vi "control_PID.vi"() -> ()   [LabVIEW 2022 SP3]
uses:
  <vilib>/Utility/NIReport.llb/Report Type.ctl
  <vilib>/imath/engines/lvmath2/RunTimeEngine/Managers/WorkSpace/UID Generator.vi
  <vilib>/imath/engines/lvmath2/RunTimeEngine/BuiltInFunctions/sin/NIMS_sin(C).vi
  <instcachedir>/0/NIMS_sin(C)_E954A9BB68A349B3841053E554BADAA4.lvgen/NIMS_sin(C)_E954A9BB68A349B3841053E554BADAA4_001.vi
  <vilib>/imath/engines/lvmath2/RunTimeEngine/BuiltInFunctions/cos/NIMS_cos(C).vi
  <instcachedir>/0/NIMS_cos(C)_24E28D29219C4DC6ABC084DC6A0254BF.lvgen/NIMS_cos(C)_24E28D29219C4DC6ABC084DC6A0254BF_001.vi
  <vilib>/imath/engines/lvmath2/RunTimeEngine/BuiltInFunctions/conv/NIMS_conv(V,V).vi
  <instcachedir>/0/NIMS_conv(V,V)_D3E194F2B5174935BB2368CEB7AAC5A9.lvgen/NIMS_conv(V,V)_D3E194F2B5174935BB2368CEB7AAC5A9_000.vi
  <vilib>/imath/engines/lvmath2/RunTimeEngine/ErrorHandling/NIMS_Error From Error Code.vi
  <vilib>/imath/engines/lvmath2/RunTimeEngine/RunTimeType/NIMS_RunTimeType_From StrictType (excl LVString).vi
  <instcachedir>/0/NIMS_RunTimeType_From StrictType (excl LVString)_70DEE8F51B6B495C85F505DE4E7061F1.lvgen/NIMS_RunTimeType_From StrictType (excl LVString)_70DEE8F51B6B495C85F505DE4E7061F1_000.vi
  <vilib>/imath/engines/lvmath2/RunTimeEngine/LocalVariableDefStatement/MC_LocalVariableDefStatement_Display.vi
  <vilib>/imath/engines/lvmath2/RunTimeEngine/IndexRead/NIMS V(S).vi
  <instcachedir>/0/NIMS V(S)_0488751826AF41519A22953C041130DC.lvgen/NIMS V(S)_0488751826AF41519A22953C041130DC_003.vi
  <vilib>/imath/engines/lvmath2/RunTimeEngine/ErrorHandling/NIMS_Create Error From Enums.vi
  <vilib>/imath/engines/lvmath2/RunTimeEngine/BuiltInFunctions/inv/NIMS_inv(GM).vi
  <instcachedir>/0/NIMS_inv(GM)_A6DF8FE880224208AACFE4CF9F659502.lvgen/NIMS_inv(GM)_A6DF8FE880224208AACFE4CF9F659502_001.vi
  <vilib>/imath/engines/lvmath2/RunTimeEngine/ArithmeticOperatorToken/NIMS_ArithmeticOperator_multmx(M,CV).vi
  <instcachedir>/0/NIMS_ArithmeticOperator_multmx(M,CV)_F5DBFFF0126A4383B39F7B34D5ABA6C8.lvgen/NIMS_ArithmeticOperator_multmx(M,CV)_F5DBFFF0126A4383B39F7B34D5ABA6C8_002.vi
  <vilib>/imath/engines/lvmath2/RunTimeEngine/IndexRead/NIMS M(S).vi
  <instcachedir>/0/NIMS M(S)_B826C018497E4940AE96BD27B540B6FB.lvgen/NIMS M(S)_B826C018497E4940AE96BD27B540B6FB_004.vi
  <vilib>/imathl/engines/lvmath/Functions/Error Handling/Create Error.vi
  <vilib>/imath/engines/lvmath2/RunTimeEngine/Managers/SymbolTable/Clear UID.vi
  <vilib>/imath/engines/lvmath2/RunTimeEngine/NodeEndStatement/NIMS_NodeEndStatement_Output.vi
  <instcachedir>/0/NIMS_NodeEndStatement_Output_53EC0D466D134D7ABD903AC30B43404B.lvgen/NIMS_NodeEndStatement_Output_53EC0D466D134D7ABD903AC30B43404B_001.vi
  <instcachedir>/0/NIMS_NodeEndStatement_Output_53EC0D466D134D7ABD903AC30B43404B.lvgen/NIMS_NodeEndStatement_Output_53EC0D466D134D7ABD903AC30B43404B_008.vi
  <vilib>/imath/engines/lvmath2/RunTimeEngine/ErrorHandling/NIMS_Finalize Error.vi
  <vilib>/addons/_office/excel.llb/Excel Easy Table (num).vi
  <vilib>/Utility/NIReport.llb/NI_report.lvclass
  <vilib>/imath/engines/lvmath2/RunTimeEngine/Managers/SymbolTable/NIMS_WorkSpace.lvlib
  <vilib>/addons/_office/NI_ReportGenerationToolkit.lvlib
  <vilib>/Utility/NIReport.llb/NI_ReportGenerationCore.lvlib
  <vilib>/Utility/NIReport.llb/Excel/NI_Excel.lvclass
panel:
  in  "Perturbacion":bool
  in  "template (empty)":path
  out "Wn":dbl
  in  "b2":dbl=0.1498
  in  "b1":dbl=0.008316
  in  "a2":dbl
  in  "a1":dbl=-0.8261
  in  "E":dbl=0.8
  in  "tss":dbl=170.0
  in  "Tm":dbl=10.0
  out "q2":dbl
  out "q1":dbl
  out "q0":dbl
  out "Graph":cluster{dbl, "SP":dbl, dbl, dbl}(graph)
  in  "SP":dbl
  in  "?":bool
  # "Condiciones \nde diseño"
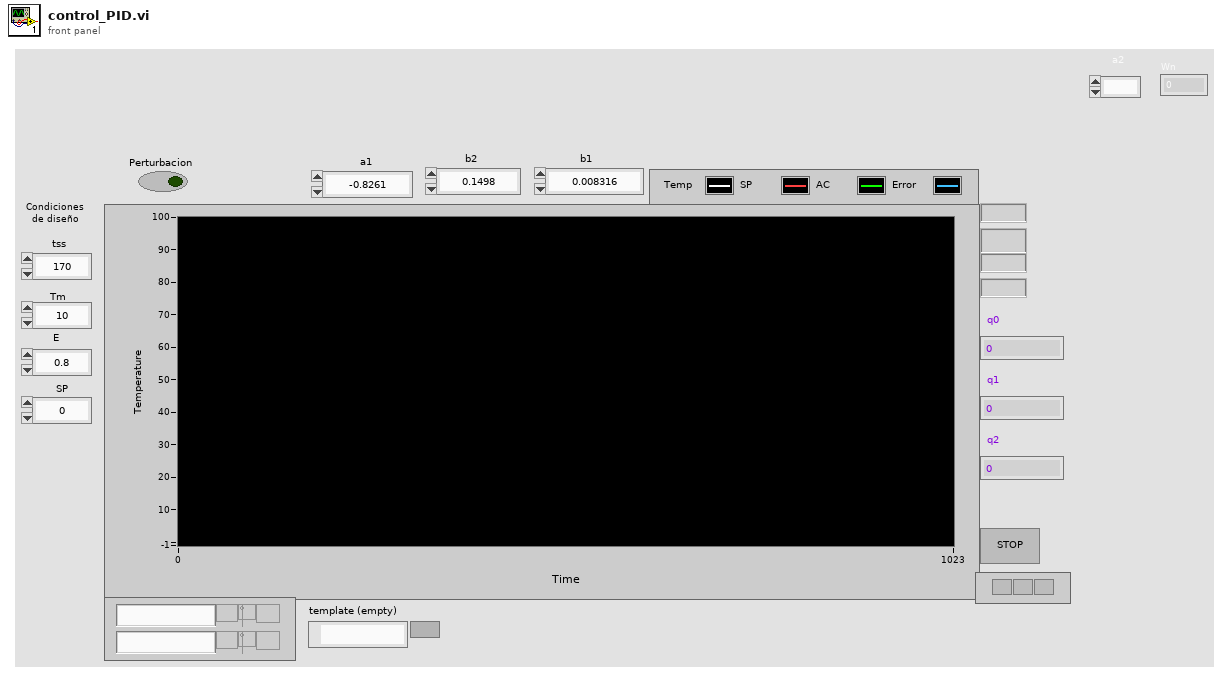
[diagram p1: front panel]
types:
  T1 = typedef "NI_ReportGenerationCore.lvlib/Report Type.ctl" = enum16{"HTML", "Word", "Excel"}
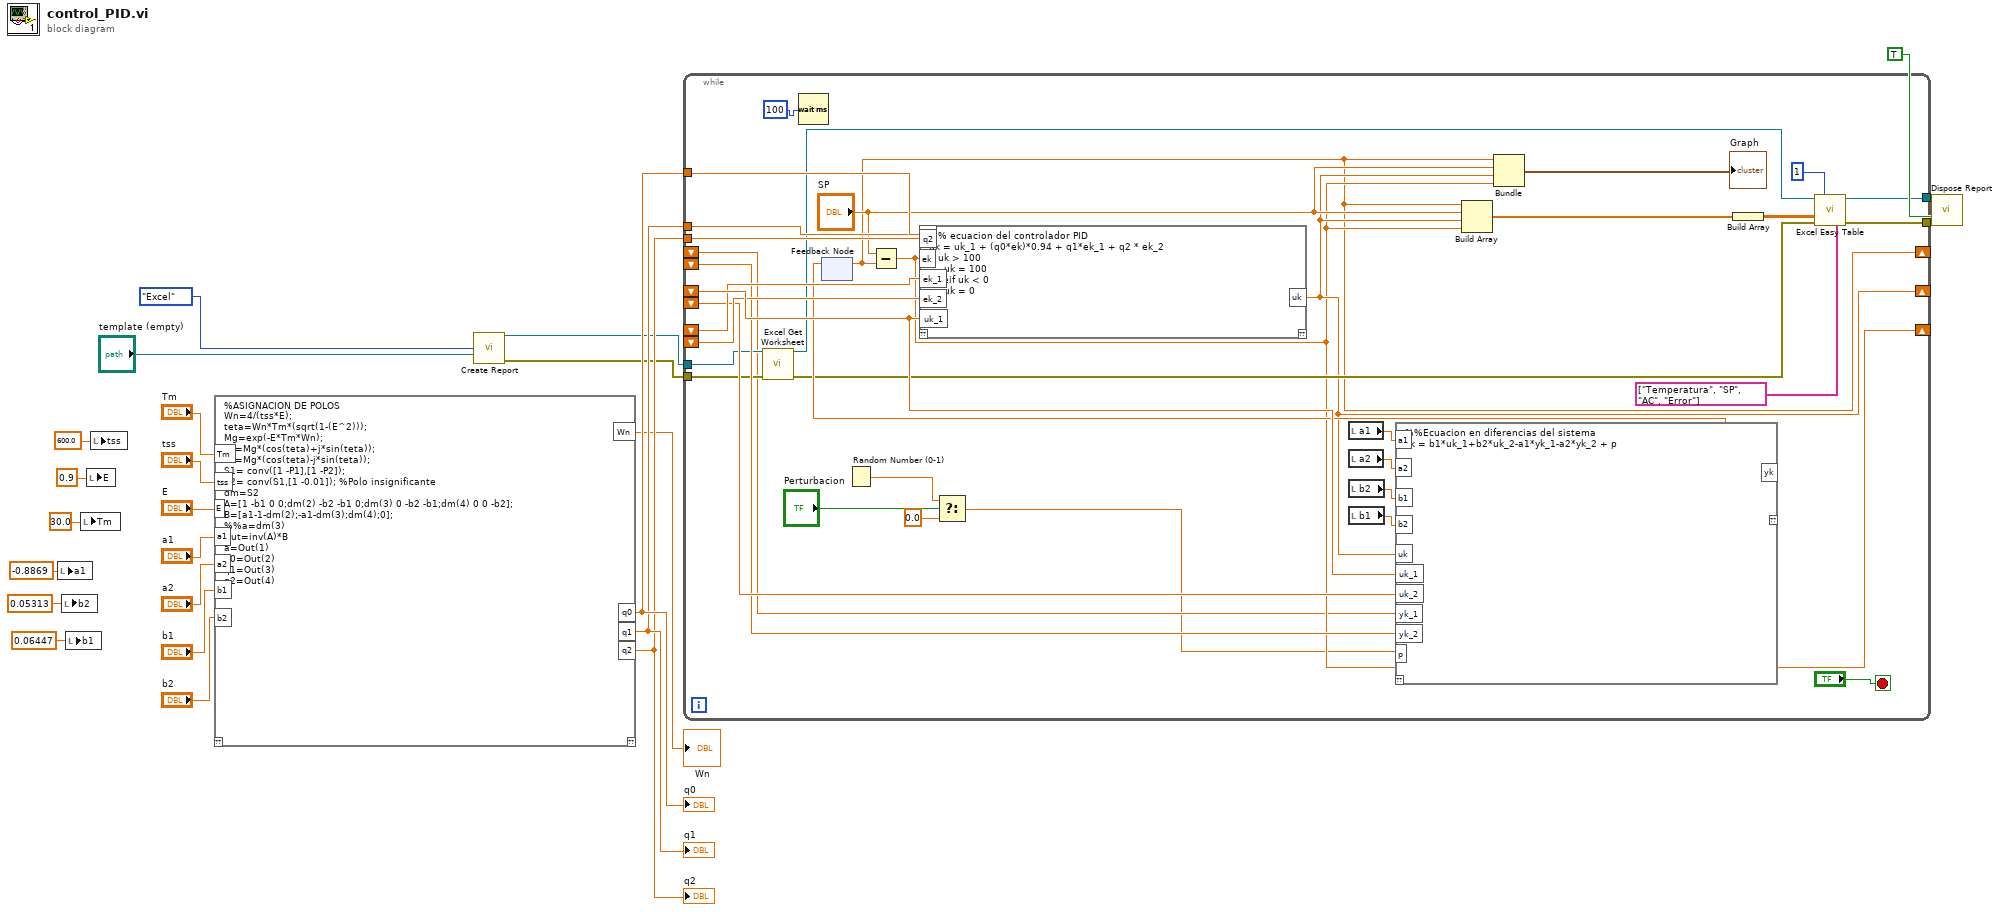
[diagram p0: block diagram]
diagram:
  n1 = local write "a1"(-0.8869 ("a1")) -> ()
  n2 = local write "b2"(0.05313 ("b2")) -> ()
  n3 = local write "b1"(0.06447 ("b1")) -> ()
  n4 = local write "Tm"(30.0 ("Tm")) -> ()
  n5 = local write "E"(0.9 ("E")) -> ()
  n6 = local write "tss"(600.0 ("tss")) -> ()
  n7 = mathscript code="%ASIGNACION DE POLOS\nWn=4/(tss*E);\nteta=Wn*Tm*(sqrt(1-(E^2)));\nMg=exp(-E*Tm*Wn);\nP1=Mg*(cos(teta)+j*sin(teta));\nP2=Mg*(cos(teta)-j*sin(teta));\nS1= conv([1 -P1],[1 -P2]);\nS2= conv(S1,[1 -0.01]); %Polo insignificante \ndm=S2\nA=[1 -b1 0 0;dm(2) -b2 -b1 0;dm(3) 0 -b2 -b1;dm(4) 0 0 -b2];\nB=[a1-1-dm(2);-a1-dm(3);dm(4);0];\n%%a=dm(3)\nOut=inv(A)*B\na=Out(1)\nq0=Out(2)\nq1=Out(3)\nq2=Out(4)"("Tm"="Tm", "tss"="tss", "E"="E", "a1"="a1", "a2"="a2", "b1"="b1", "b2"="b2") -> ("q0"=w24:cdb, "q1"=w23:cdb, "q2"=w22:cdb, "Wn"=→"Wn":dbl)  [unwired: 1 in, 1 out]
  "q0" <- w24
  "q1" <- w23
  "q2" <- w22
  n8 = call <vilib>:"Create Report.vi"("report type"=Report_Type."Excel", "template (empty)"="template (empty)") -> ("report out"=w10:refnum<class "NI_report.lvclass">, "error out"=w9:errorcluster)  [unwired: 12 in]
  n9 = while {
    shift-right: [w30] -> _
    shift-left: _ -> [w31]
    tunnel: w24 -> [w58]
    tunnel: w23 -> [w57]
    tunnel: w22 -> [w56]
    shift-right: [w35] -> _
    shift-left: _ -> [w54]
    shift-left: _ -> [w53]
    shift-right: [w36] -> _
    shift-left: _ -> [w55]
    shift-left: _ -> [w51]
    shift-left: _ -> [w50]
    tunnel: w10 -> [w41]
    tunnel: w9 -> [w40]
    tunnel: [w39] -> w8
    tunnel: [w38] -> w7
    stop <- "?" stop-if-true
    n10 = call <vilib>:"Excel Get Worksheet.vi"("report in"=w41, "error in (no error)"=w40) -> ("report out"=w45:refnum<class "NI_report.lvclass">, "error out"=w44:errorcluster)  [unwired: 12 in]
    n11 = Wait (ms)(milliseconds to wait=u32 100) -> ()  [unwired: 1 out]
    n12 = feedback #1() -> (w30:cdb)  [unwired: 1 in]
    n13 = Random Number (0-1)() -> (number: 0 to 1=w27:dbl)
    n14 = Subtract(x="SP", y=w30) -> (x-y=w35:cdb)
    n15 = mathscript code="%% ecuacion del controlador PID\nuk = uk_1 + (q0*ek)*0.94 + q1*ek_1 + q2 * ek_2\nif uk > 100\n     uk = 100\nelseif uk < 0\n     uk = 0 \nend"("q0"=w58, "q1"=w57, "q2"=w56, "ek"=w35, "ek_1"=w54, "ek_2"=w53, "uk_1"=w55) -> ("uk"=w36:cdb)  [unwired: 1 in, 1 out]
    n16 = Select(t=w27, s="Perturbacion", f=0.0) -> (s? t:f=w26:dbl)
    n17 = local read "a1"() -> (w49:dbl)
    n18 = local read "a2"() -> (w48:dbl)
    n19 = local read "b2"() -> (w47:dbl)
    n20 = local read "b1"() -> (w46:dbl)
    n21 = mathscript code="%%Ecuacion en diferencias del sistema\nyk = b1*uk_1+b2*uk_2-a1*yk_1-a2*yk_2 + p"("uk"=w36, "uk_1"=w55, "yk_1"=w31, "uk_2"=w51, "a1"=w49, "a2"=w48, "b1"=w47, "b2"=w46, "yk_2"=w50, "p"=w26) -> ("yk"=w52:cdb)  [unwired: 1 in, 1 out]
    n22 = feedback-in #1(w52) -> ()
    n23 = Build Array(w30, "SP", w36, w35) -> (w34:cdb[])
    n24 = Bundle("yk"=w30, "SP"="SP", "uk"=w36, w35) -> (→"Graph":cluster{"yk":cdb, "SP":dbl, "uk":cdb, cdb})  [unwired: 1 in]
    n25 = Build Array(w34) -> (w43:cdb[][])
    n26 = call-poly <vilib>:"Excel Easy Table.vi"("report in"=w45, "iteration"=1, "text data"=w43, "error in (no error)"=w44, "column headers"=string[] ["Temperatura", "SP", "AC", "Error"]) -> ("report out"=w39:refnum<class "NI_report.lvclass">, "error out"=w38:errorcluster)  [unwired: 6 in, 3 out]
  }
  n27 = call-dynamic "Dispose Report.vi"("report in"=w8, "save changes? (F)"=TRUE, "error in (no error)"=w7) -> ()  [unwired: 12 in, 1 out]
